vi "Read Cource OutputOffset.vi"(8 "error in (no error)":errorcluster, 11 "BME_DG_G08_Chnl in":refnum<class "BME_DG_G08_Chnl.lvclass">) -> (0 "error out":errorcluster, 2 "Cource OutputOffset":bool=TRUE, 3 "BME_DG_G08_Chnl out":refnum<class "BME_DG_G08_Chnl.lvclass">)   [LabVIEW 2009, in "POLARIS BME DG.lvlib" / "BME_DG_G08_Chnl.lvclass"]
uses:
  BME_DG_G08_Chnl.lvclass
  BME_DG_G08_Chnl.lvclass/BME_DG_G08_Chnl.ctl
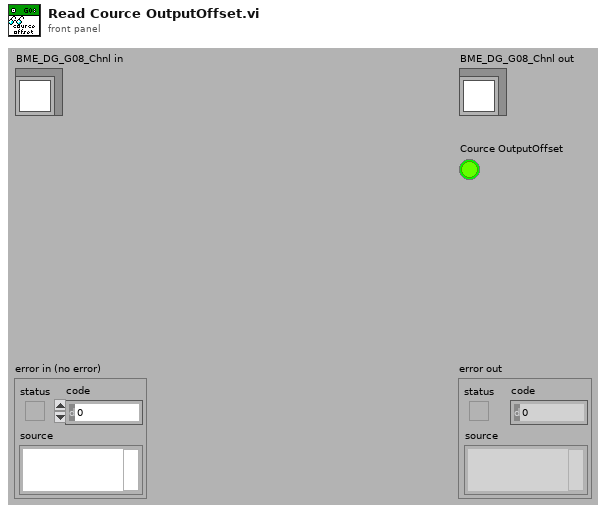
[diagram p1: front panel]
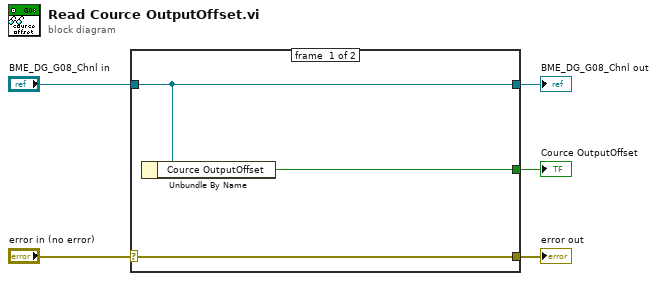
[diagram p0: block diagram]
diagram:
  n1 = case shown="No Error" "error in (no error)" {
    selector: "error in (no error)" -> [w8 w9]
    tunnel: [w8 w9] -> w4
    tunnel: [w7 w10] -> w2
    tunnel: "BME_DG_G08_Chnl in" -> [w7 w10]
    tunnel: [w6 _] -> w1
    frame #0 {
      n2 = Unbundle By Name(w7) -> ("Cource OutputOffset"=w6:bool)
    }
    frame #1 {
    }
  }
  "error out" <- w4
  "BME_DG_G08_Chnl out" <- w2
  "Cource OutputOffset" <- w1
